vi "PSU_close.vi"(11 "VISA resource name":refnum<visa-resource-name>) -> ()   [LabVIEW 2023]
uses:
  <instrlib>/BK Precision 91xx Series/BK Precision 91xx Series.lvlib
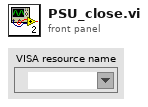
[diagram p1: front panel]
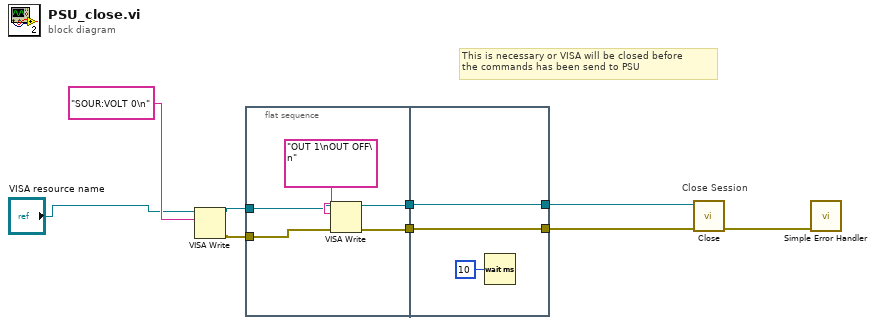
[diagram p0: block diagram]
diagram:
  # "This is necessary or VISA will be closed before\nthe commands has been send to PSU"
  # "Close Session"
  n1 = VISA Write(VISA resource name="VISA resource name", write buffer="SOUR:VOLT 0\n" ("format string")) -> (VISA resource name out=w4:refnum<visa-resource-name>, error out=w3:errorcluster)  [unwired: 1 in, 1 out]
  n2 = flat-sequence {
    tunnel: w4 -> [w11]
    tunnel: w3 -> [w10]
    tunnel: [w12] -> w2
    tunnel: [w13] -> w1
    tunnel: [w16] -> w7
    tunnel: [w17] -> w8
    tunnel: w2 -> [w17]
    tunnel: w1 -> [w16]
    frame #0 {
      n3 = VISA Write(VISA resource name=w11, write buffer="OUT 1\nOUT OFF\n", error in (no error)=w10) -> (VISA resource name out=w12:refnum<visa-resource-name>, error out=w13:errorcluster)  [unwired: 1 out]
    }
    frame #1 {
      n4 = Wait (ms)(milliseconds to wait=u32 10) -> ()  [unwired: 1 out]
    }
  }
  n5 = call <instrlib>:"Close.vi"("error in (no error)"=w7, "VISA resource name"=w8) -> ("error out"=w9:errorcluster)  [unwired: 9 in]
  n6 = call <vilib>:"Simple Error Handler.vi"("error in (no error)"=w9) -> ()  [unwired: 4 in, 5 out]
